vi "Hahn Plus RF sweep Pulse Sequence Generator.vi"(0 "Pulse offset":dbl, 5 "Array":T1(array[cluster]), 6 "MW Delay":dbl, 7 "No. Instructions":i32, 9 "Tau":dbl, 10 "RF Pulse":dbl, 11 "Rabi Frequency":dbl) -> (3 "Pulse Sequence":T1(array[cluster]))   [LabVIEW 2012]
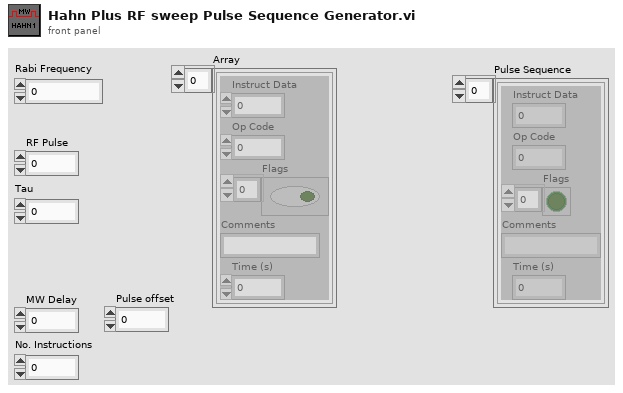
[diagram p1: front panel]
types:
  T1 = cluster{"Instruct Data":i32, "Op Code":i32, "Flags":bool[], "Comments":string, "Time (s)":dbl}[]
  T2 = cluster{"Instruct Data":i32, "Op Code":i32, "Flags":bool[], "Comments":string, "Time (s)":dbl}
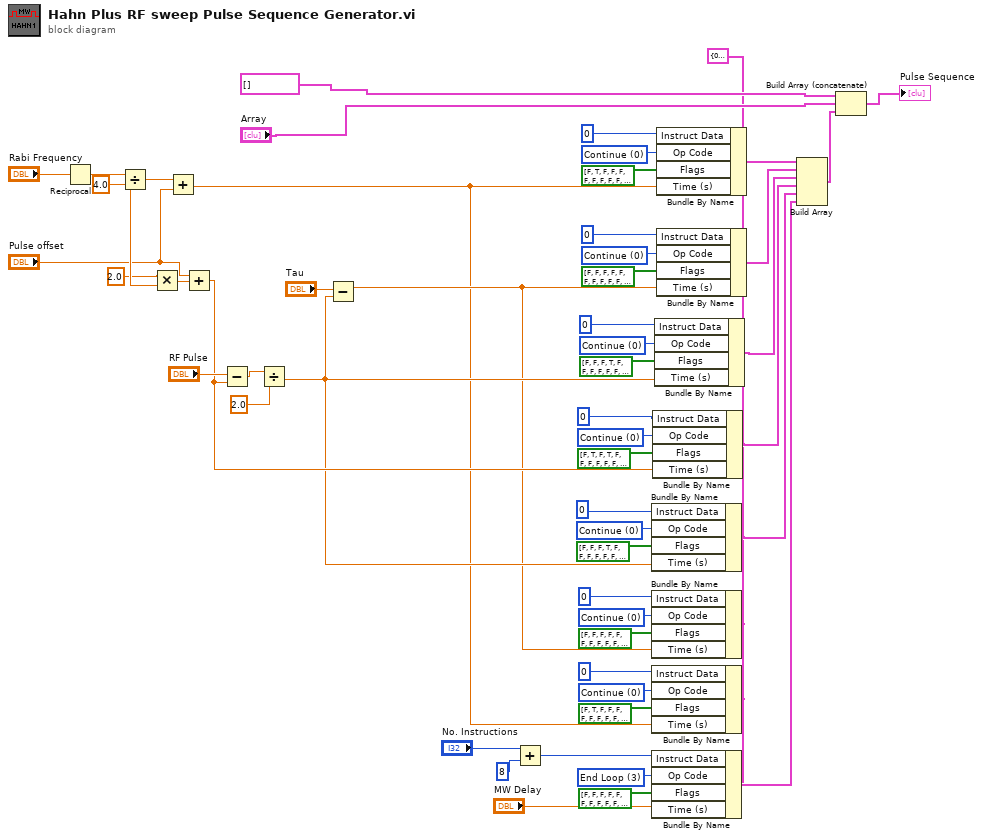
[diagram p0: block diagram]
diagram:
  w7 = 0 items=["Continue", "Stop", "Loop", "End Loop", "JSR", "RTS", "Branch", "Long Delay", "Wait"] ("Op Code")
  w10 = 0 items=["Continue", "Stop", "Loop", "End Loop", "JSR", "RTS", "Branch", "Long Delay", "Wait"] ("Op Code")
  w27 = 3 items=["Continue", "Stop", "Loop", "End Loop", "JSR", "RTS", "Branch", "Long Delay", "Wait"] ("Op Code")
  w30 = 0 items=["Continue", "Stop", "Loop", "End Loop", "JSR", "RTS", "Branch", "Long Delay", "Wait"] ("Op Code")
  w33 = 0 items=["Continue", "Stop", "Loop", "End Loop", "JSR", "RTS", "Branch", "Long Delay", "Wait"] ("Op Code")
  w37 = 0 items=["Continue", "Stop", "Loop", "End Loop", "JSR", "RTS", "Branch", "Long Delay", "Wait"] ("Op Code")
  w40 = 0 items=["Continue", "Stop", "Loop", "End Loop", "JSR", "RTS", "Branch", "Long Delay", "Wait"] ("Op Code")
  w43 = 0 items=["Continue", "Stop", "Loop", "End Loop", "JSR", "RTS", "Branch", "Long Delay", "Wait"] ("Op Code")
  w5 = T2 {"Instruct Data"=0, "Op Code"=0, "Flags"=[FALSE, FALSE, FALSE, FALSE, FALSE, FALSE, FALSE, FALSE, FALSE, FALSE, FALSE, FALSE, FALSE, FALSE, FALSE, FALSE, FALSE, FALSE, FALSE, FALSE, FALSE, TRUE, TRUE, TRUE], "Comments"="", "Time (s)"=0.01} ("PB Inst 2")
  n1 = Reciprocal(x="Rabi Frequency") -> (1/x=w52:dbl)
  n2 = Divide(x=w52, y=4.0) -> (x/y=w51:dbl)
  n3 = Multiply(x=2.0, y=w51) -> (x*y=w35:dbl)
  n4 = Add(x=w51, y="Pulse offset") -> (x+y=w3:dbl)
  n5 = Add(x="Pulse offset", y=w35) -> (x+y=w13:dbl)
  n6 = Subtract(x="RF Pulse", y=w13) -> (x-y=w16:dbl)
  n7 = Divide(x=w16, y=2.0) -> (x/y=w12:dbl)
  n8 = Subtract(x="Tau", y=w12) -> (x-y=w4:dbl)
  n9 = Add(x="No. Instructions", y=8) -> (x+y=w2:i32)
  n10 = Bundle By Name(cluster=w5, "Instruct Data"=0, "Op Code"=w30, "Flags"=bool[] [FALSE, FALSE, FALSE, TRUE, FALSE, FALSE, FALSE, FALSE, FALSE, FALSE, FALSE, FALSE, FALSE, FALSE, FALSE, FALSE, FALSE, FALSE, FALSE, FALSE, FALSE, TRUE, TRUE, TRUE], "Time (s)"=w12) -> (w22:T2)
  n11 = Bundle By Name(cluster=w5, "Instruct Data"=0, "Op Code"=w10, "Flags"=bool[] [FALSE, FALSE, FALSE, FALSE, FALSE, FALSE, FALSE, FALSE, FALSE, FALSE, FALSE, FALSE, FALSE, FALSE, FALSE, FALSE, FALSE, FALSE, FALSE, FALSE, FALSE, TRUE, TRUE, TRUE], "Time (s)"=w4) -> ()  [unwired: 1 out]
  n12 = Bundle By Name(cluster=w5, "Instruct Data"=0, "Op Code"=w7, "Flags"=bool[] [FALSE, TRUE, FALSE, FALSE, FALSE, FALSE, FALSE, FALSE, FALSE, FALSE, FALSE, FALSE, FALSE, FALSE, FALSE, FALSE, FALSE, FALSE, FALSE, FALSE, FALSE, TRUE, TRUE, TRUE], "Time (s)"=w3) -> ()  [unwired: 1 out]
  n13 = Bundle By Name(cluster=w5, "Instruct Data"=w2, "Op Code"=w27, "Flags"=bool[] [FALSE, FALSE, FALSE, FALSE, FALSE, FALSE, FALSE, FALSE, FALSE, FALSE, FALSE, FALSE, FALSE, FALSE, FALSE, FALSE, FALSE, FALSE, FALSE, FALSE, FALSE, TRUE, TRUE, TRUE], "Time (s)"="MW Delay") -> (w23:T2)
  n14 = Bundle By Name(cluster=w5, "Instruct Data"=0, "Op Code"=w33, "Flags"=bool[] [FALSE, TRUE, FALSE, TRUE, FALSE, FALSE, FALSE, FALSE, FALSE, FALSE, FALSE, FALSE, FALSE, FALSE, FALSE, FALSE, FALSE, FALSE, FALSE, FALSE, FALSE, TRUE, TRUE, TRUE], "Time (s)"=w13) -> (w21:T2)
  n15 = Bundle By Name(cluster=w5, "Instruct Data"=0, "Op Code"=w37, "Flags"=bool[] [FALSE, FALSE, FALSE, TRUE, FALSE, FALSE, FALSE, FALSE, FALSE, FALSE, FALSE, FALSE, FALSE, FALSE, FALSE, FALSE, FALSE, FALSE, FALSE, FALSE, FALSE, TRUE, TRUE, TRUE], "Time (s)"=w12) -> (w20:T2)
  n16 = Bundle By Name(cluster=w5, "Instruct Data"=0, "Op Code"=w43, "Flags"=bool[] [FALSE, TRUE, FALSE, FALSE, FALSE, FALSE, FALSE, FALSE, FALSE, FALSE, FALSE, FALSE, FALSE, FALSE, FALSE, FALSE, FALSE, FALSE, FALSE, FALSE, FALSE, TRUE, TRUE, TRUE], "Time (s)"=w3) -> (w24:T2)
  n17 = Bundle By Name(cluster=w5, "Instruct Data"=0, "Op Code"=w40, "Flags"=bool[] [FALSE, FALSE, FALSE, FALSE, FALSE, FALSE, FALSE, FALSE, FALSE, FALSE, FALSE, FALSE, FALSE, FALSE, FALSE, FALSE, FALSE, FALSE, FALSE, FALSE, FALSE, TRUE, TRUE, TRUE], "Time (s)"=w4) -> (w19:T2)
  n18 = Build Array(w24, w19, w20, w21, w22, w23) -> (w25:T1)
  n19 = Build Array (concatenate)(T1 [], "Array", w25) -> (→"Pulse Sequence":T1)
